vi "CommandDynamixelPosition.vi"(8 "Error in":errorcluster, 10 "Sail settings":T1 {"MainSailSuggestion" min=0.0 max=1.0; "JibSailSuggestion" min=0.0 max=1.0}, 11 "VISA UART port":refnum<visa-resource-name>) -> (0 "Error out":errorcluster)   [LabVIEW 2013]
uses:
  Data/TypeDefs/Sail Set Suggestions.ctl
panel:
  out "return count":u32
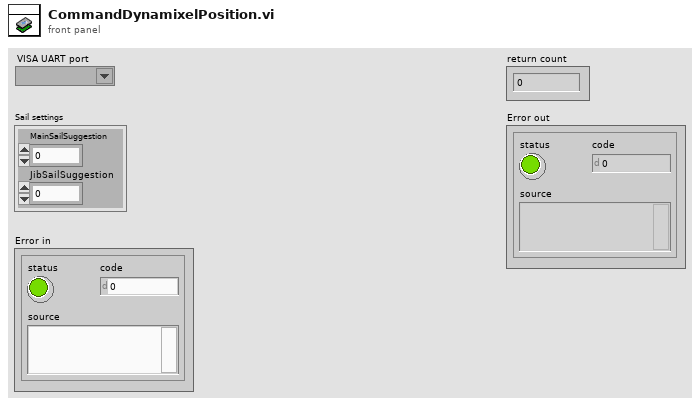
[diagram p1: front panel]
types:
  T1 = typedef "Sail Set Suggestions.ctl" = cluster{"MainSailSuggestion":dbl, "JibSailSuggestion":dbl}
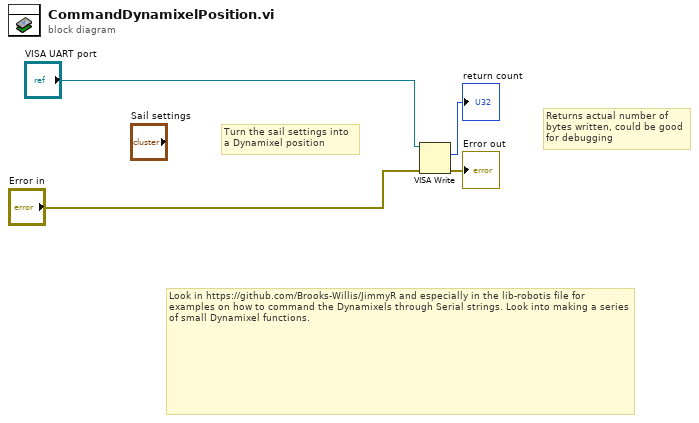
[diagram p0: block diagram]
diagram:
  # "Turn the sail settings into a Dynamixel position"
  # "Returns actual number of bytes written, could be good for debugging"
  # "Look in https://github.com/Brooks-Willis/JimmyR and especially in the lib-robotis file for examples on how to command the Dynamixels through Serial strings. Look into making a series of small Dynamixel functions."
  n1 = VISA Write(VISA resource name="VISA UART port", error in (no error)="Error in") -> (return count=→"return count":u32, error out=→"Error out":errorcluster)  [unwired: 1 in, 1 out]
